vi "Entity Definition.vi"(11 "Entity in":refnum<class "Entity.lvclass">) -> (2 "Definition":refnum<class "Type.lvclass">[](array[class]))   [LabVIEW 2020, in "Conditu2.lvlib" / "Entity.lvclass"]
uses:
  Entity.lvclass
  Columns/Type/Type.lvclass
  Columns/ID/ID.lvclass
  C:/dev/lv20CE/lv-conditum-tools/Conditum-Clone/Columns/Type/Type.lvclass
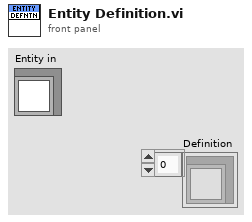
[diagram p1: front panel]
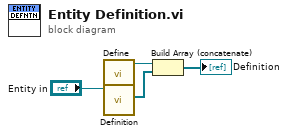
[diagram p0: block diagram]
diagram:
  n1 = call "Define.vi"() -> ("ID out"=w3:refnum<class "ID.lvclass">)  [unwired: 11 in]
  n2 = call-dynamic "Definition.vi"("Entity"="Entity in") -> ("Entity Definition"=w2:refnum<class "Type.lvclass">[])  [unwired: 10 in]
  n3 = Build Array (concatenate)(w3, w2) -> (→"Definition":refnum<class "Type.lvclass">[])
